vi "update_dict_HIS_work.vi"(8 "error in (no error)":errorcluster, 9 "Control":string="+1", 10 "type":string, 11 "dict of HIS IN":variant) -> (0 "error out":errorcluster, 3 "dict of HIS OUT":variant)   [LabVIEW 2015]
uses:
  cluster_template.ctl
  Classes/DATA/HIS/HIS.lvclass
  Classes/DATA/DATA.lvclass/DATA.ctl
  Classes/DATA/HIS/HIS.lvclass/HIS.ctl
  Classes/DATA/DATA.lvclass
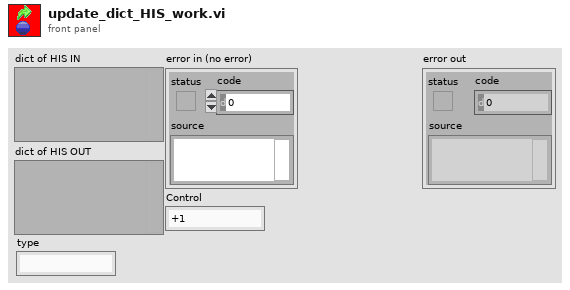
[diagram p1: front panel]
types:
  T1 = typedef "cluster_template.ctl" = cluster{"HIS.lvclass":refnum<class "HIS.lvclass">, "selector":refnum<vi>, "HIS graph":refnum<vi>, "DAT graph":refnum<vi>, "path":refnum<vi>, "path MAIN":refnum<vi>, "#":refnum<vi>, "unsel Graph":refnum<vi>, "DATgraph":refnum<vi>}
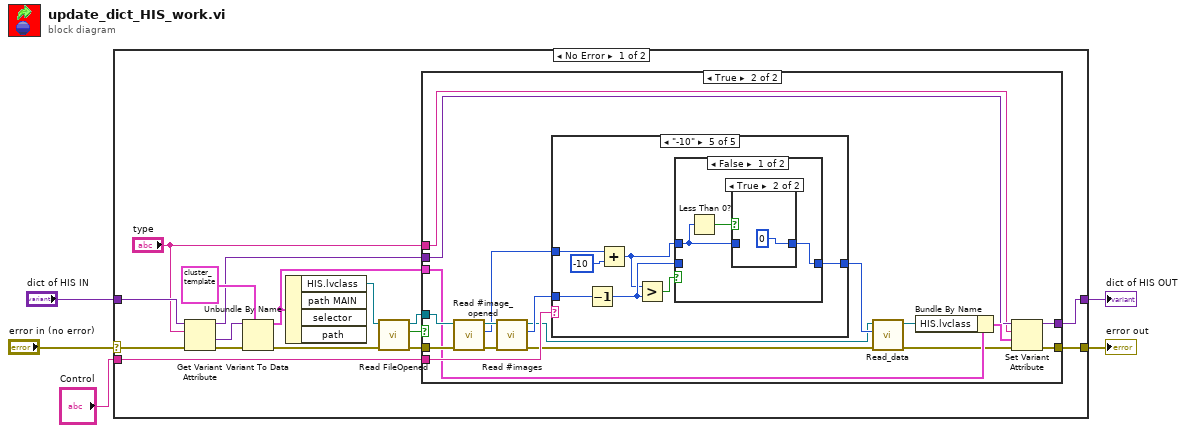
[diagram p0: block diagram]
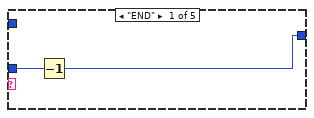
[diagram p3: hidden frame]
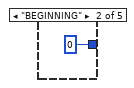
[diagram p4: hidden frame]
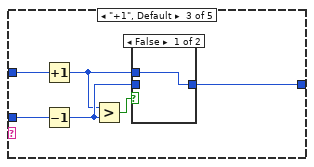
[diagram p5: hidden frame]
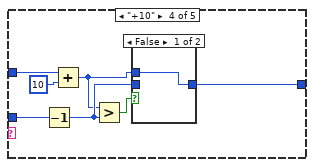
[diagram p7: hidden frame]
diagram:
  n1 = case shown="No Error" "error in (no error)" {
    selector: "error in (no error)" -> [w20 w76]
    tunnel: "dict of HIS IN" -> [w21 w75]
    tunnel: [w9 w75] -> w4
    tunnel: [w7 w76] -> w3
    tunnel: "Control" -> [w12 _]
    frame No Error {
      n2 = Get Variant Attribute(Variant=w21, name="type", error in=w20) -> (duplicate Variant=w8:variant, value=w19:variant, error out=w18:errorcluster)  [unwired: 1 in, 1 out]
      n3 = Variant To Data(error in=w18, type=T1 {"HIS.lvclass"=refnum, "selector"=refnum, "HIS graph"=refnum, "DAT graph"=refnum, "path"=refnum, "path MAIN"=refnum, "#"=refnum, "unsel Graph"=refnum, "DATgraph"=refnum} ("output cluster"), Variant=w19) -> (data=w10:T1, error out=w15:errorcluster)
      n4 = Unbundle By Name(w10) -> ("HIS.lvclass"=w16:refnum<class "HIS.lvclass">)  [unwired: 3 out]
      n5 = call "Read FileOpened.vi"("error in (no error)"=w15, "DATA in"=w16) -> ("error out"=w11:errorcluster, "FileOpened"=w14:bool, "DATA out"=w13:refnum<class "HIS.lvclass">)  [unwired: 7 in]
      n6 = case shown="True" w14 {
        tunnel: w13 -> [_ w41]
        tunnel: w12 -> [_ w40]
        tunnel: w11 -> [w23 w35]
        tunnel: [w23 w27] -> w7
        tunnel: w10 -> [_ w29]
        tunnel: [w22 w26] -> w9
        tunnel: w8 -> [w22 w25]
        tunnel: "type" -> [_ w24]
        frame False {
        }
        frame True {
          n7 = call "Read #image_opened.vi"("error in (no error)"=w35, "HIS in"=w41) -> ("error out"=w39:errorcluster, "#image_opened"=w32:i32, "HIS out"=w38:refnum<class "HIS.lvclass">)  [unwired: 7 in]
          n8 = call "Read #images.vi"("error in (no error)"=w39, "HIS in"=w38) -> ("error out"=w34:errorcluster, "#images"=w37:i32, "HIS out"=w33:refnum<class "HIS.lvclass">)  [unwired: 7 in]
          n9 = case shown="\"-10\"" w40 {
            tunnel: [w42 0 w47 w57 w66] -> w36
            tunnel: w37 -> [w43 _ w49 w59 w68]
            tunnel: w32 -> [_ _ w50 w55 w64]
            frame "END" {
              n10 = Decrement(x=w43) -> (x-1=w42:i32)
            }
            frame "BEGINNING" {
            }
            frame "+1", Default {
              n11 = Increment(x=w50) -> (x+1=w45:i32)
              n12 = Decrement(x=w49) -> (x-1=w46:i32)
              n13 = Greater?(x=w45, y=w46) -> (0:w48:bool)
              n14 = case shown="False" w48 {
                tunnel: [w51 w52] -> w47
                tunnel: w46 -> [_ w52]
                tunnel: w45 -> [w51 _]
                frame False {
                }
                frame True {
                }
              }
            }
            frame "+10" {
              n15 = Decrement(x=w59) -> (x-1=w56:i32)
              n16 = Add(x=w55, y=10) -> (x+y=w54:i32)
              n17 = Greater?(x=w54, y=w56) -> (0:w58:bool)
              n18 = case shown="False" w58 {
                tunnel: [w60 w61] -> w57
                tunnel: w56 -> [_ w61]
                tunnel: w54 -> [w60 _]
                frame False {
                }
                frame True {
                }
              }
            }
            frame "-10" {
              n19 = Decrement(x=w68) -> (x-1=w65:i32)
              n20 = Add(x=w64, y=-10) -> (x+y=w63:i32)
              n21 = Greater?(x=w63, y=w65) -> (0:w67:bool)
              n22 = case shown="False" w67 {
                tunnel: [w69 w74] -> w66
                tunnel: w65 -> [_ w74]
                tunnel: w63 -> [w70 _]
                frame False {
                  n23 = Less Than 0?(x=w70) -> (x < 0?=w71:bool)
                  n24 = case shown="True" w71 {
                    tunnel: w70 -> [w72 _]
                    tunnel: [w72 0] -> w69
                    frame False {
                    }
                    frame True {
                    }
                  }
                }
                frame True {
                }
              }
            }
          }
          n25 = call-dynamic "Read_data.vi"("error in (no error)"=w34, "#image"=w36, "HIS IN"=w33) -> ("error out"=w28:errorcluster, "HIS OUT"=w30:refnum<class "HIS.lvclass">)  [unwired: 7 in]
          n26 = Bundle By Name(cluster=w29, "HIS.lvclass"=w30) -> (w31:T1)
          n27 = Set Variant Attribute(Variant=w25, name=w24, value=w31, error in=w28) -> (Variant out=w26:variant, error out=w27:errorcluster)  [unwired: 1 out]
        }
      }
    }
    frame Error {
    }
  }
  "dict of HIS OUT" <- w4
  "error out" <- w3
